vi "SubVI_ConnectToSingle.vi"(8 "error in (no error)":errorcluster, 11 "Path":path) -> (0 "error out":errorcluster, 1 "Write":string, 2 "Read":string, 3 "Handle":u32 format="%x")   [LabVIEW 2023, in "ADS_Library.lvlib"]
doc: "This VI is designed to be the first in a set of VIs used to read/write symbols from TwinCAT.\nThis VI takes a string with a single symbol for a read or write operation.\nIt then creates the connection for the choosen symbol, this can then be passed to the SingleSymbolRead or SingleSymbolWrite VIs"
uses:
  ADS_Library.lvlib
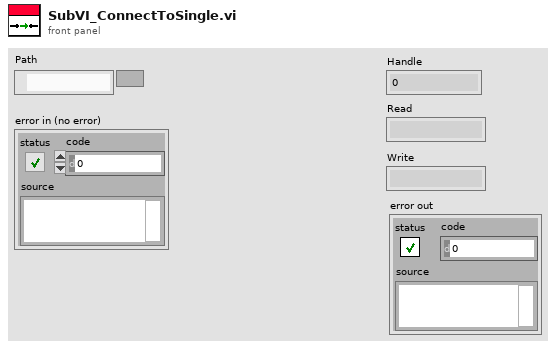
[diagram p1: front panel]
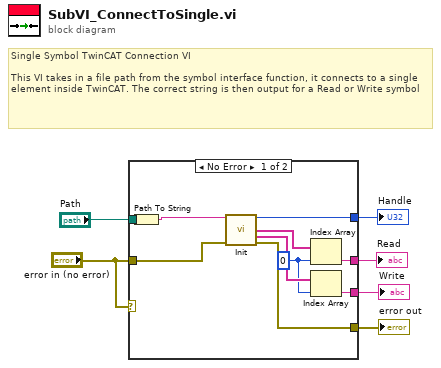
[diagram p0: block diagram]
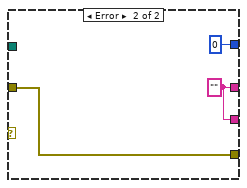
[diagram p2: hidden frame]
diagram:
  # "Single Symbol TwinCAT Connection VI\n\nThis VI takes in a file path from the symbol interface function, it connects to a single element inside TwinCAT. The correct string is then output for a Read or Write symbol"
  n1 = case shown="No Error" "error in (no error)" {
    tunnel: "Path" -> [w16 _]
    tunnel: "error in (no error)" -> [w14 w19]
    tunnel: [w13 u32 0 ("Handle")] -> w5
    tunnel: [w10 w19] -> w4
    tunnel: [w8 w18] -> w3
    tunnel: [w7 w18] -> w2
    frame No Error {
      w9 = 0 ("index")
      n2 = Path To String(path=w16) -> (string=w15:string)
      n3 = call <userlib>:"Init.vi"("XMLDescription"=w15, "error in (no error)"=w14) -> ("Handle"=w13:u32, "ReadGrpSymbols"=w12:string[], "WriteGrpSymbols"=w11:string[], "error out"=w10:errorcluster)  [unwired: 9 in, 1 out]
      n4 = Index Array(array=w12, index=w9) -> (element=w8:string)
      n5 = Index Array(array=w11, index=w9) -> (element=w7:string)
    }
    frame Error {
      w18 = "" ("ReadGrpSymbols")
    }
  }
  "Handle" <- w5
  "error out" <- w4
  "Read" <- w3
  "Write" <- w2
